vi "retrieve_polarity_values.vi"(5 "Error In":errorcluster) -> (19 "Error Out":errorcluster)   [LabVIEW 2013, in "examples.lvlib"]
doc: "Retrieve all the current polarity values at the specified axis. For single-axis applications, the axis input need not be specified.\n\nProduced By:\n\n<B>Kod Integrations, LLC</B>\n4835 Marianne Drive\nMount Airy, MD 21771\nhttp://www.kodintegrations.com\nemail: info@kodintegrations.com\nphone: (240) 687-1288"
uses:
  libraries/examples.lvlib
  classes/Controller/_Controller.lvclass
  common/controls/axis.ctl
  libraries/common.lvlib
  common/controls/polarity.ctl
  common/controls/polarity_item.ctl
panel:
  out "polarity_items (out)":T1[](array[typedef])
  in  "axis (def=X)":T3
  in  "clear_buffer? (T)":bool=TRUE
  in  "device_index (in) [0=def]":i32
  # "instructions:\n\nFor single-axis applications simply specify the device\nindex and run the VI.  For multi-axis applications,\nspecify both the device index and the controller\naxis, then run the VI"
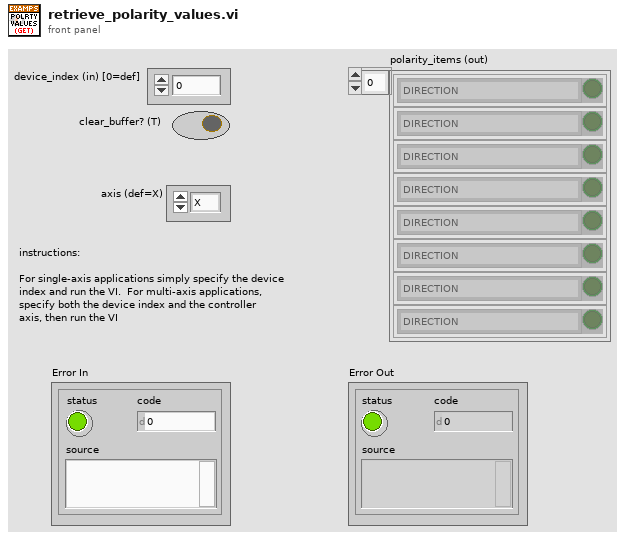
[diagram p1: front panel]
types:
  T1 = typedef "common.lvlib/polarity_item.ctl" = cluster{"item":T2, "status":bool}
  T2 = typedef "common.lvlib/polarity.ctl" = enum16{"DIRECTION", "LIMIT", "HOME", "DIG_OUT", "DIG_IN", "ENABLE_OUT", "JUMP_ERR", "LATCH", "Z-CHAN_INDEX", "ENCODER_DECODING:1X", "ENCODER_DECODING:2X", "ENCODER_DECODING:4X", "ALARM", "STANDALONE_ERR", "-", "<reserved/nc>"}
  T3 = typedef "common.lvlib/axis.ctl" = enum16{"X", "Y", "Z", "U"}
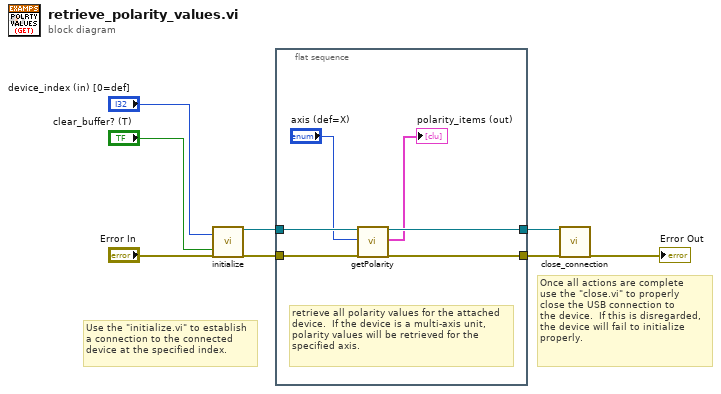
[diagram p0: block diagram]
diagram:
  # "Once all actions are complete\nuse the \"close.vi\" to properly\nclose the USB connection to \nthe device.  If this is disregarded,\nthe device will fail to initialize \nproperly."
  # "Use the \"initialize.vi\" to establish\na connection to the connected\ndevice at the specified index."
  n1 = call "initialize.vi"("device_index (in) [0=def]"="device_index (in) [0=def]", "clear_buffer? (T)"="clear_buffer? (T)", "error in (no error)"="Error In") -> ("reference (out)"=w5:refnum<class "_Controller.lvclass">, "error out"=w4:errorcluster)  [unwired: 15 in]
  n2 = flat-sequence {
    tunnel: w5 -> [w14]
    tunnel: w4 -> [w13]
    tunnel: [w11] -> w3
    tunnel: [w12] -> w2
    frame #0 {
      # "retrieve all polarity values for the attached\ndevice.  If the device is a multi-axis unit,\npolarity values will be retrieved for the\nspecified axis."
      n3 = call-dynamic "getPolarity.vi"("Controller in"=w14, "axis (def=X)"="axis (def=X)", "error in (no error)"=w13) -> ("Controller out"=w11:refnum<class "_Controller.lvclass">, "polarity_items (out)"=→"polarity_items (out)":T1[], "error out"=w12:errorcluster)  [unwired: 14 in]
    }
  }
  n4 = call "close_connection.vi"("reference (in)"=w3, "error in (no error)"=w2) -> ("error out"=→"Error Out":errorcluster)  [unwired: 16 in, 1 out]
